vi "BSCAN_DEMO07_v2_Zynq_DDR3_MT41K.vi"() -> ()   [LabVIEW 2017]
uses:
  Saldigi_protocol_library.lvlibp
panel:
  out "dt":dbl=0.6003044999961276
  in  "stop":bool
  out "test mask OK":bool=TRUE
  in  "Data bus width":enum16{"16bit Data bus", "32bit Data bus"}(ring)=enum."32bit Data bus"
  out "error out":errorcluster
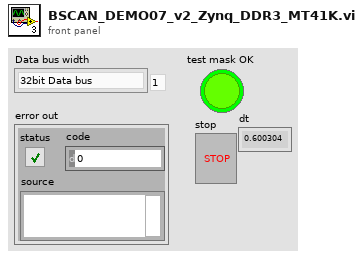
[diagram p1: front panel]
types:
  T1 = typedef "Saldigi_protocol_library.lvlibp/DDR3_BSCAN_typedef.ctl" = cluster{"DDR3 PORTs aliases":string[], "DDR3 PORTs BSCAN init states":bool[], "DDR3 PORTs BSCAN indexes":u32[], "DDR3 PORTs ControlCell BSCAN indexes":u32[], "DDR3 PORTs ControlCell BSCAN safe state":bool[], "DDR3 bidir PORTs ControlCell relativeIndex":u32[], "DDR3 bidir PORTs ControlCell relativeIndex safe state":bool[], "CKP PORT alias":string, "CKN PORT alias":string, "DDR3 Address [15-14:0] input array length":i32, "DDR3 Data [NN:0] input array length":i32, "DDR3 Bank[2:0] input array length\nCKP\nCKN":i32, "DDR3 Clocking Strobe input array length":i32, "DDR3 CKE CS# RAS# CAS# WE#(LSB) input array length":i32, "DDR3 Constant input array length":i32, "DDR3 PORTs ReadCell BSCAN indexes":u32[]}
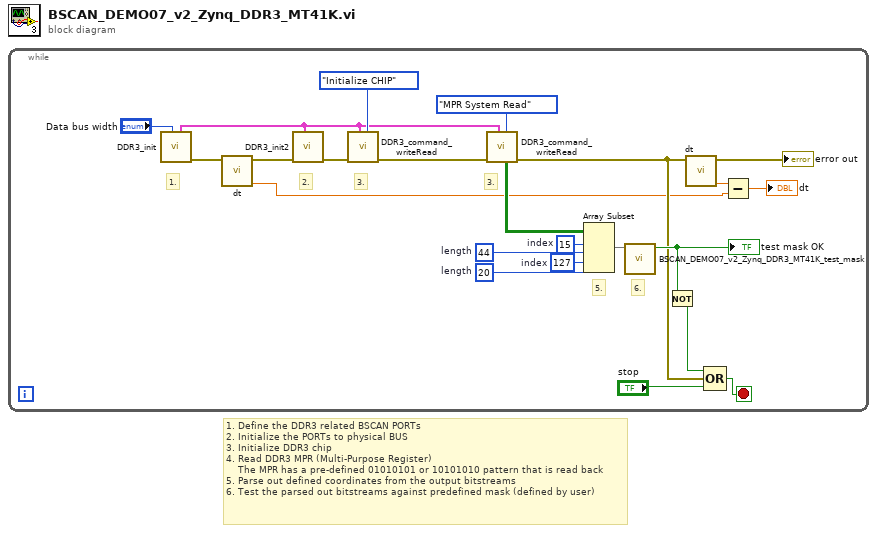
[diagram p0: block diagram]
diagram:
  # "1. Define the DDR3 related BSCAN PORTs\n2. Initialize the PORTs to physical BUS\n3. Initialize DDR3 chip\n4. Read DDR3 MPR (Multi-Purpose Register)\n    The MPR has a pre-defined 01010101 or 10101010 pattern that is read back\n5. Parse out defined coordinates from the output bitstreams\n6. Test the parsed out bitstreams against predefined mask (defined by user)"
  n1 = while {
    stop <- w9 stop-if-true
    w15 = 20  # length
    w16 = 127  # index
    w17 = 44  # length
    w18 = 15  # index
    # "6."
    # "5."
    # "3."
    # "3."
    # "2."
    # "1."
    n2 = call "DDR3_init.vi"("Data bus width"="Data bus width") -> ("error out"=w7:errorcluster, "DDR3 BSCAN typedef out"=w20:T1)  [unwired: 9 in]
    n3 = call "dt.vi"("error in"=w7) -> ("relative seconds"=w4:dbl, "error out"=w6:errorcluster)  [unwired: 9 in]
    n4 = call "DDR3_init2.vi"("DDR3 BSCAN typedef"=w20, "error in"=w6) -> ("error out"=w23:errorcluster)  [unwired: 9 in]
    n5 = call "DDR3_command_writeRead.vi"("Enum"=enum16{"Initialize CHIP", "MPR System Read"}."Initialize CHIP", "DDR3 BSCAN typedef in"=w20, "error in"=w23) -> ("error out"=w19:errorcluster)  [unwired: 7 in, 1 out]
    n6 = call "DDR3_command_writeRead.vi"("Enum"=enum16{"Initialize CHIP", "MPR System Read"}."MPR System Read", "DDR3 BSCAN typedef in"=w20, "error in"=w19) -> ("error out"=w8:errorcluster, "read data out"=w12:bool[][])  [unwired: 7 in]
    n7 = Array Subset(array=w12, index (row)=w18, length (row)=w17, index (col)=w16, length (col)=w15) -> (w14:bool[][])
    n8 = call "BSCAN_DEMO07_v2_Zynq_DDR3_MT41K_test_mask.vi"("Test read data out"=w14) -> ("test mask OK"=w11:bool)  [unwired: 10 in]
    "test mask OK" <- w11
    n9 = Not(x=w11) -> (.not. x?=w2:bool)
    n10 = call "dt.vi"("error in"=w8) -> ("relative seconds"=w5:dbl, "error out"=→"error out":errorcluster)  [unwired: 9 in]
    n11 = Compound Arithmetic op=OR(w2, w8, "stop") -> (w9:bool)
    n12 = Subtract(x=w5, y=w4) -> (x-y=→"dt":dbl)
  }
